vi "via xml report.vi"(8 "error in (no error)":errorcluster, 10 "Path":path, 11 "Analysis Results":T9 {"Test Config Data"."Test Ranking" items=["Low", "Normal", "High"]}) -> (0 "error out":errorcluster)   [LabVIEW 2014, in "VIA-Checkstyle.lvlib"]
doc: "Saves VI Analzyer test results in an XML format compatible with Checkstyle static code analysis reports."
uses:
  VIA-Checkstyle.lvlib
  <vilib>/addons/analyzer/_analyzerctrls.llb/VIAnCtl Results.ctl
  <vilib>/addons/analyzer/_analyzerctrls.llb/VIAnCtl ResultsData (index).ctl
  <vilib>/addons/analyzer/_analyzerctrls.llb/VIAnCtl ResultStatus.ctl
  <vilib>/addons/analyzer/_vianresshared.llb/VIAnRes Parsed Results Data (by VI).ctl
  <vilib>/addons/analyzer/_vianresshared.llb/VIAnRes Parsed Results Data (by Test).ctl
  <vilib>/addons/analyzer/_analyzerctrls.llb/VIAnCtl Test Config Data.ctl
  <vilib>/addons/analyzer/_analyzerctrls.llb/VIAnCtl TestRanking.ctl
  <vilib>/addons/analyzer/_analyzerctrls.llb/VIAnCtl Config Control Value.ctl
  xml format - file.ctl
  xml format - error.ctl
panel:
  out "serialized results":string
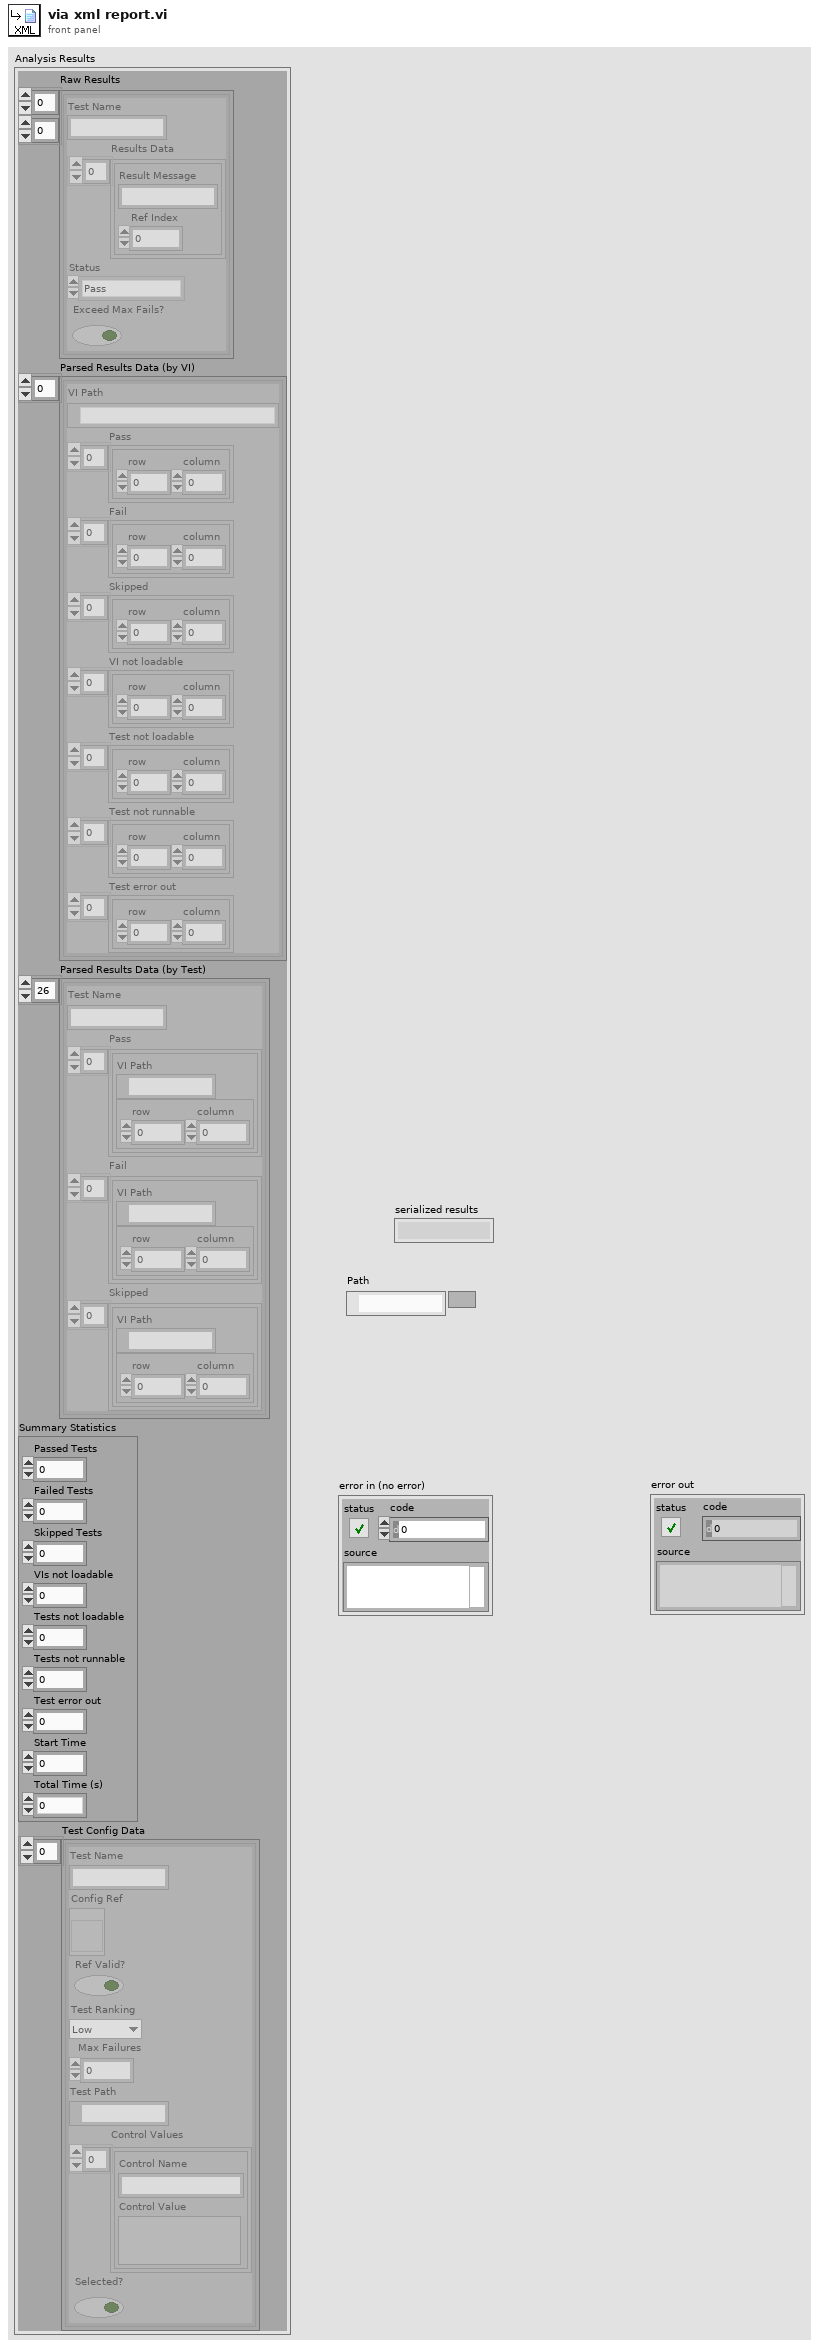
[diagram p1: front panel]
types:
  T1 = typedef "VIAnCtl Results.ctl" = cluster{"Test Name":string, "Results Data":T2[], "Status":T3, "Exceed Max Fails?":bool}
  T2 = typedef "VIAnCtl ResultsData (index).ctl" = cluster{"Result Message":string, "Ref Index":i32}
  T3 = typedef "VIAnCtl ResultStatus.ctl" = enum16{"Pass", "Fail", "Skipped", "VI not loadable", "Test not loadable", "Test not runnable", "Test error out"}
  T4 = typedef "VIAnRes Parsed Results Data (by VI).ctl" = cluster{"VI Path":path, "Pass":cluster{"row":i32, "column":i32}[], "Fail":cluster{"row":i32, "column":i32}[], "Skipped":cluster{"row":i32, "column":i32}[], "VI not loadable":cluster{"row":i32, "column":i32}[], "Test not loadable":cluster{"row":i32, "column":i32}[], "Test not runnable":cluster{"row":i32, "column":i32}[], "Test error out":cluster{"row":i32, "column":i32}[]}
  T5 = typedef "VIAnRes Parsed Results Data (by Test).ctl" = cluster{"Test Name":string, "Pass":cluster{"VI Path":path, "index":cluster{"row":i32, "column":i32}}[], "Fail":cluster{"VI Path":path, "index":cluster{"row":i32, "column":i32}}[], "Skipped":cluster{"VI Path":path, "index":cluster{"row":i32, "column":i32}}[]}
  T6 = typedef "VIAnCtl Test Config Data.ctl" = cluster{"Test Name":string, "Config Ref":refnum<vi>, "Ref Valid?":bool, "Test Ranking":T7, "Max Failures":u32, "Test Path":path, "Control Values":T8[], "Selected?":bool}
  T7 = typedef "VIAnCtl TestRanking.ctl" = u16
  T8 = typedef "VIAnCtl Config Control Value.ctl" = cluster{"Control Name":string, "Control Value":variant}
  T9 = cluster{"Raw Results":T1[][], "Parsed Results Data (by VI)":T4[], "Parsed Results Data (by Test)":T5[], "Summary Statistics":cluster{"Passed Tests":i32, "Failed Tests":i32, "Skipped Tests":i32, "VIs not loadable":i32, "Tests not loadable":i32, "Tests not runnable":i32, "Test error out":i32, "Start Time":u32, "Total Time (s)":dbl}, "Test Config Data":T6[]}
  T10 = enum16{"open", "replace", "create", "open or create", "replace or create", "replace or create with confirmation"}
  T11 = typedef "VIA-Checkstyle.lvlib/xml format - error.ctl" = cluster{"severity":enum16{"info", "warning", "error"}, "message":string, "source":string, "row":i32, "column":i32}
  T12 = typedef "VIA-Checkstyle.lvlib/xml format - file.ctl" = cluster{"errors":T11[], "name":string}
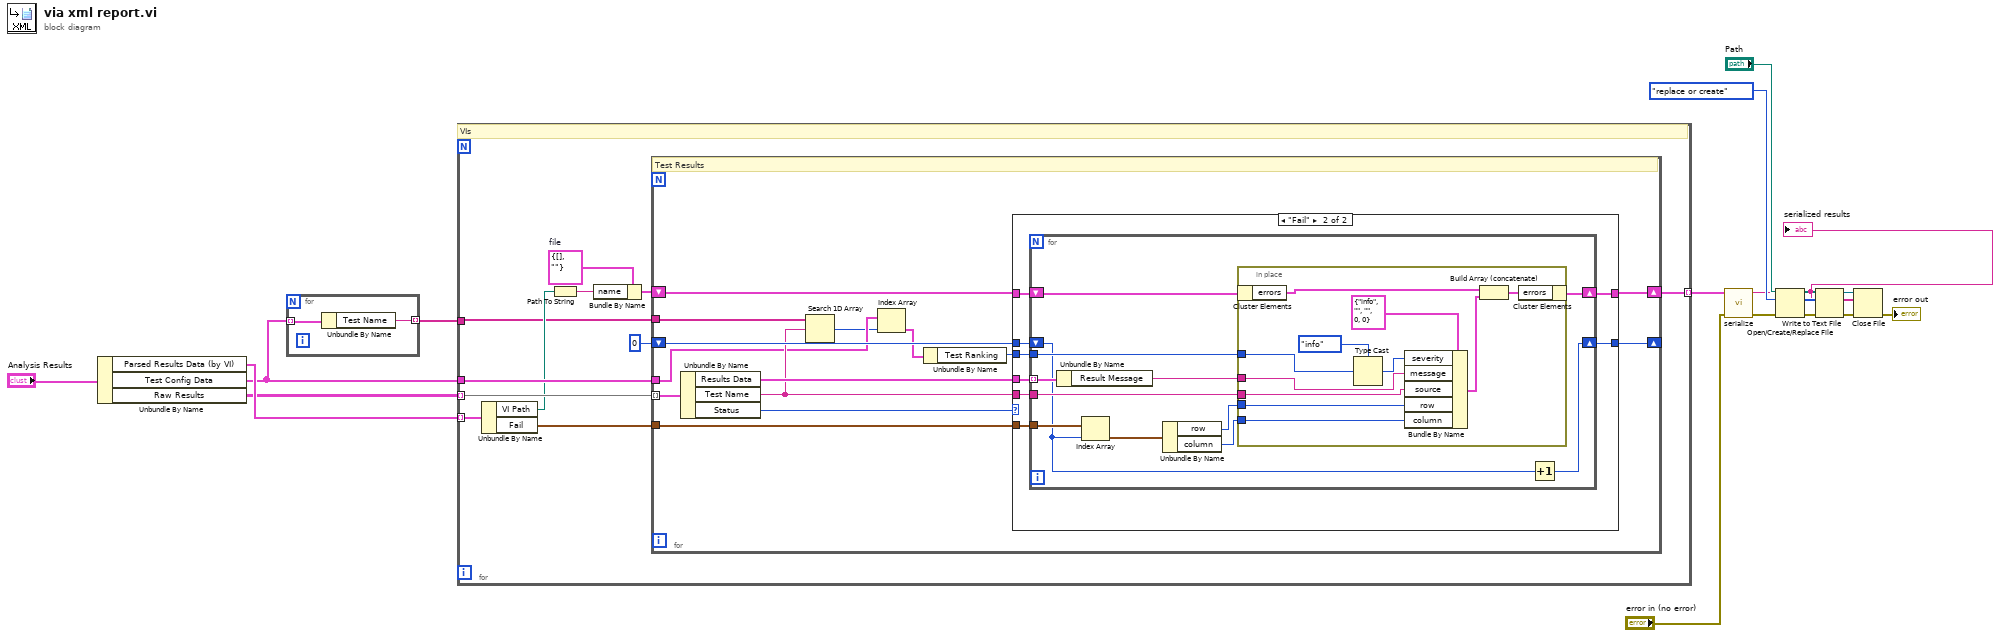
[diagram p0: block diagram]
diagram:
  n1 = Unbundle By Name("Analysis Results") -> ("Parsed Results Data (by VI)"=w15:T4[], "Test Config Data"=w2:T6[], "Raw Results"=w14:T1[][])
  n2 = for {
    tunnel: w2 -> [w18] mode=indexing
    tunnel: [w17] -> w1 mode=indexing
    n3 = Unbundle By Name(w18) -> ("Test Name"=w17:string)
  }
  n4 = for {
    tunnel: w14 -> [w29] mode=indexing
    tunnel: w2 -> [w28]
    tunnel: w15 -> [w26] mode=indexing
    tunnel: [w20] -> w13 mode=indexing
    tunnel: w1 -> [w19]
    w27 = T12 {"errors"=[], "name"=""}  # file
    # "VIs"
    n5 = Unbundle By Name(w26) -> ("VI Path"=w25:path, "Fail"=w22:cluster{"row":i32, "column":i32}[])
    n6 = Path To String(path=w25) -> (string=w24:string)
    n7 = Bundle By Name(cluster=w27, "name"=w24) -> (w23:T12)
    n8 = for {
      tunnel: w29 -> [w43] mode=indexing
      tunnel: w28 -> [w32]
      shift-right: [w40] -> w20
      shift-left: w23 -> [w42]
      tunnel: w22 -> [w37]
      shift-right: [w35] -> _
      shift-left: 0 -> [w36]
      tunnel: w19 -> [w34]
      # "Test Results"
      n9 = Unbundle By Name(w43) -> ("Results Data"=w39:T2[], "Test Name"=w33:string, "Status"=w38:T3)
      n10 = Search 1D Array(1D array=w34, element=w33) -> (index of element=w31:i32)  [unwired: 1 in]
      n11 = Index Array(array=w32, index=w31) -> (element=w30:T6)
      n12 = Unbundle By Name(w30) -> ("Test Ranking"=w41:T7)
      n13 = case shown="\"Fail\"" w38 {
        tunnel: w42 -> [w45 w53]
        tunnel: w33 -> [_ w52]
        tunnel: w41 -> [_ w51]
        tunnel: [w45 w50] -> w40
        tunnel: w39 -> [_ w49]
        tunnel: w37 -> [_ w48]
        tunnel: w36 -> [w44 w47]
        tunnel: [w44 w46] -> w35
        frame Default {
        }
        frame "Fail" {
          n14 = for {
            tunnel: w52 -> [w64]
            tunnel: w51 -> [w63]
            shift-right: [w61] -> w50
            shift-left: w53 -> [w65]
            tunnel: w49 -> [w60] mode=indexing
            tunnel: w48 -> [w59]
            shift-right: [w54] -> w46
            shift-left: w47 -> [w55]
            n15 = Unbundle By Name(w60) -> ("Result Message"=w62:string)
            n16 = Index Array(array=w59, index=w55) -> (element=w58:cluster{"row":i32, "column":i32})
            n17 = Unbundle By Name(w58) -> ("row"=w57:i32, "column"=w56:i32)
            n18 = in-place {
              in-place-border: w64 -> [w73]
              in-place-border: w63 -> [w71]
              in-place-border: w62 -> [w69]
              in-place-border: w57 -> [w67]
              in-place-border: w56 -> [w66]
              n19 = in-place-cluster #1(w65) -> ("errors"=w76:T11[])
              n20 = Type Cast(type=enum16{"info", "warning", "error"}."info" ("severity"), x=w71) -> (*(type *) &x=w70:enum16{"info", "warning", "error"})
              n21 = Bundle By Name(cluster=T11 {"severity"=enum."info", "message"="", "source"="", "row"=0, "column"=0} ("error"), "severity"=w70, "message"=w69, "source"=w73, "row"=w67, "column"=w66) -> (w68:T11)
              n22 = Build Array (concatenate)(w76, w68) -> (w75:T11[])
              n23 = in-place-cluster #1("errors"=w75) -> (w61:T12)
            }
            n24 = Increment(x=w55) -> (x+1=w54:i32)
          }
        }
      }
    }
  }
  n25 = call "serialize.vi"("error in"="error in (no error)", "Results"=w13) -> ("error out"=w11:errorcluster, "serialized results"=w7:string)  [unwired: 8 in]
  "serialized results" <- w7
  n26 = Open/Create/Replace File(file path (use dialog)="Path", error in=w11, operation (0:open)=T10."replace or create") -> (refnum out=w8:refnum<file>, error out=w6:errorcluster)  [unwired: 3 in, 1 out]
  n27 = Write to Text File(file (use dialog)=w8, text=w7, error in=w6) -> (refnum out=w4:refnum<file>, error out=w5:errorcluster)  [unwired: 1 in, 1 out]
  n28 = Close File(refnum=w4, error in=w5) -> (error out=→"error out":errorcluster)  [unwired: 1 out]
